vi "trace_property_sub.vi"(0 "traces_spectrum":cluster{"idx":u32}[](array[cluster]), 1 "traces_interferogram":T2(array[cluster]), 5 "trace idx":u32, 7 "Strings enum":string[](array[string]), 9 "Value enum":u16, 11 "error in (no error)":errorcluster, 12 "all string":string="all_stringParameters", 14 "dataType":T1) -> (4 "global trace idx":u32, 6 "parameter names":string[](array[string]), 8 "char nr max":i32[](array[numeric]), 15 "error out":errorcluster)   [LabVIEW 2010, in "OSA.lvclass"]
uses:
  OSA.lvclass
  typeDef/acq_dataType.ctl
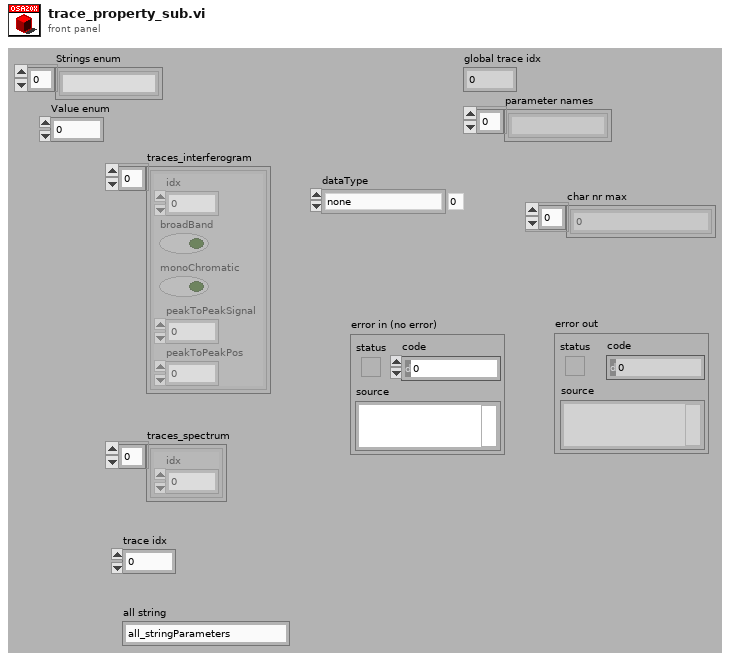
[diagram p1: front panel]
types:
  T1 = typedef "OSA.lvclass/acq_dataType.ctl" = enum16{"none", "interferogram", "spectrum"}
  T2 = cluster{"idx":u32, "broadBand":bool, "monoChromatic":bool, "peakToPeakSignal":dbl, "peakToPeakPos":dbl}[]
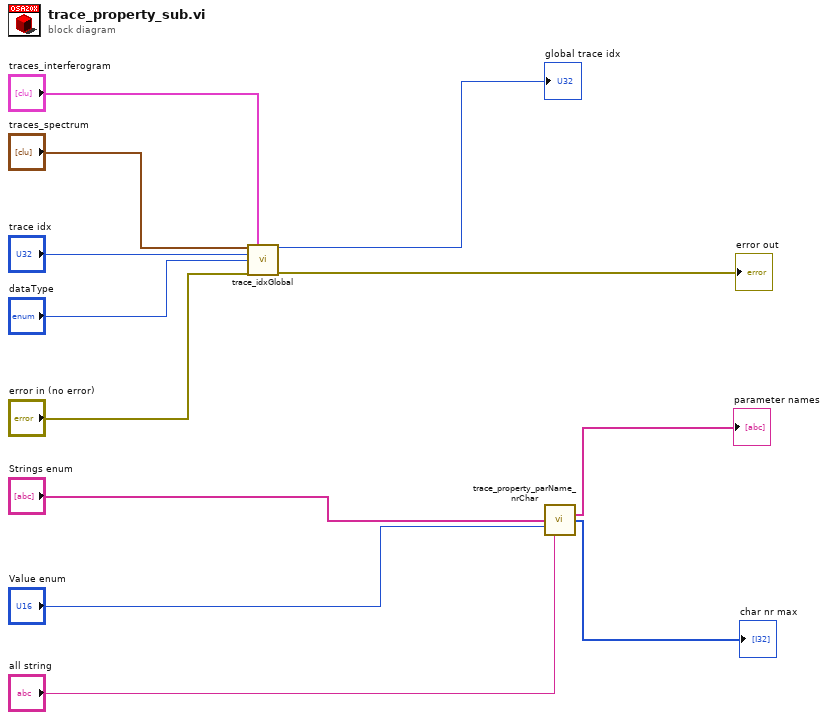
[diagram p0: block diagram]
diagram:
  n1 = call "trace_idxGlobal.vi"("traces_spectrum"="traces_spectrum", "traces_interferogram"="traces_interferogram", "trace idx"="trace idx", "dataType"="dataType", "error in (no error)"="error in (no error)") -> ("global trace idx"=→"global trace idx":u32, "error out"=→"error out":errorcluster)  [unwired: 9 in]
  n2 = call "trace_property_parName_nrChar.vi"("Strings enum"="Strings enum", "Value enum"="Value enum", "all string"="all string") -> ("parameter names"=→"parameter names":string[], "char nr max"=→"char nr max":i32[])  [unwired: 11 in]
